vi "Mirao52e.vi"() -> ()   [LabVIEW 2011]
panel:
  in  "?":enum32{"Main", "Debug"}(tab)
  in  "Flat Shape File Path":string="FLAT_MIRAO_0229_01.mro"
  out "error out":errorcluster
  out "flat":dbl[](array[numeric])
  out "received":dbl[](array[numeric])
  out "SyncString":string
  in  "Debug":bool
  out "# messages received":u64
  out "DM response":i8
  out "open return value":i8
  in  "stop":bool
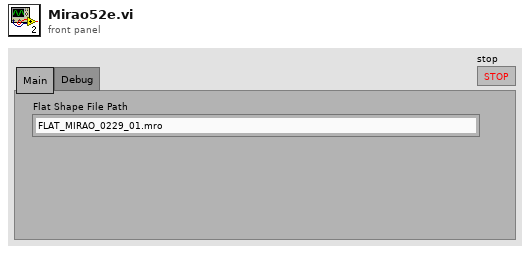
[diagram p1: front panel]
types:
  T1 = enum32{"invalid app kind", "Development System", "Run Time System", "Student Edition", "Embedded LabVIEW", "Evaluation", "Custom"}
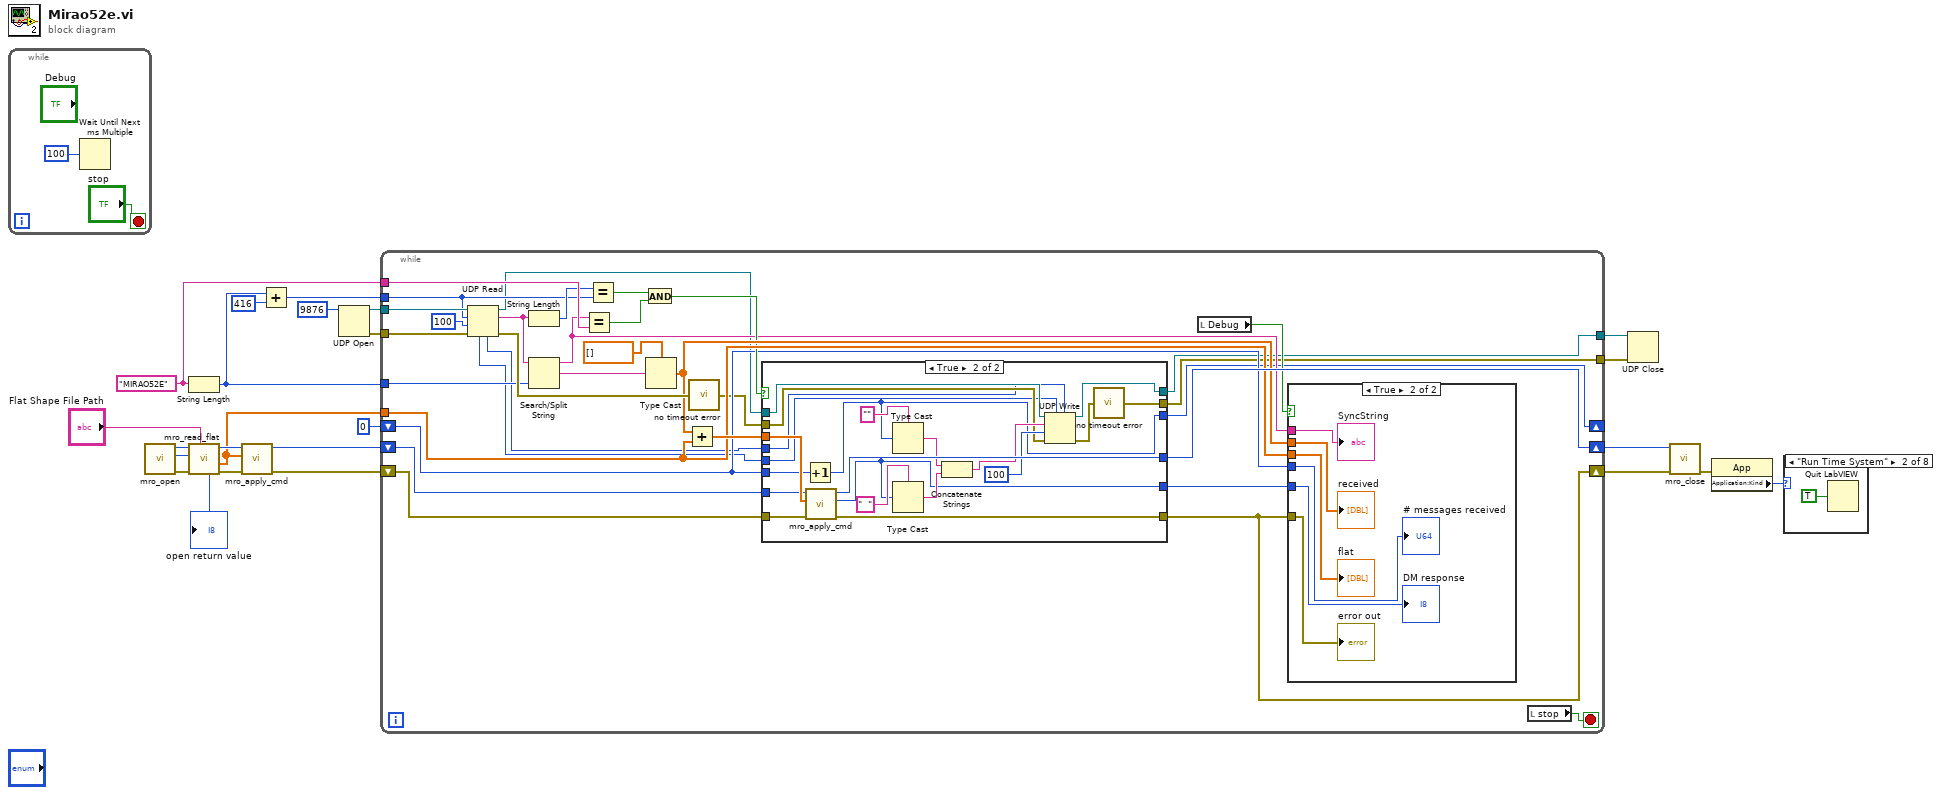
[diagram p0: block diagram]
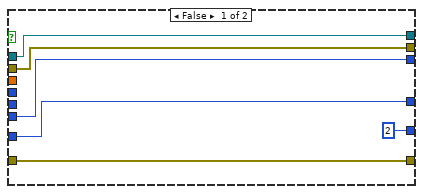
[diagram p10: hidden frame]
diagram:
  w2 = "MIRAO52E" ("data out")
  n1 = while {
    stop <- "stop" stop-if-true
    n2 = Wait Until Next ms Multiple(millisecond multiple=u32 100) -> ()  [unwired: 1 out]
  }
  n3 = call "mro_open.vi"() -> ("error out"=w21:errorcluster, "return type"=→"open return value":i8, "status"=w23:i32)  [unwired: 9 in]
  n4 = String Length(string=w2) -> (length=w3:i32)
  n5 = call "mro_read_flat.vi"("FilePath"="Flat Shape File Path", "error in (no error)"=w21, "status in"=w23) -> ("error out"=w11:errorcluster, "flat"=w9:dbl[], "status out"=w13:i32)  [unwired: 5 in, 1 out]
  n6 = call "mro_apply_cmd.vi"("error in (no error)"=w11, "command"=w9, "status in"=w13) -> ("error out"=w10:errorcluster, "status out"=w12:i32)  [unwired: 6 in, 1 out]
  n7 = Add(x=w3, y=416 ("max size (548)")) -> (x+y=w4:i32)
  n8 = UDP Open(11:u16 9876 ("Port")) -> (port=w20:refnum<k16>, 0:w19:errorcluster)  [unwired: 4 in, 1 out]
  n9 = while {
    tunnel: w9 -> [w48]
    tunnel: w20 -> [w57]
    tunnel: w19 -> [w56]
    tunnel: [w29] -> w18
    tunnel: [w30] -> w17
    shift-right: [w58] -> w22
    shift-left: w12 -> [w52]
    shift-right: [w41] -> w8
    shift-left: w10 -> [w51]
    shift-right: [w33] -> _
    shift-left: u64 0 ("Port") -> [w34]
    tunnel: w4 -> [w42]
    tunnel: w3 -> [w40]
    tunnel: w2 -> [w47]
    stop <- w35 stop-if-true
    n10 = UDP Read(connection ID=w57, max size (548)=w42, timeout ms (25000)=100, 8:w56) -> (data out=w39:string, error out=w54:errorcluster, 3:w28:refnum<k16>, 4:w26:u16, 6:w27:u32)
    n11 = String Length(string=w39) -> (length=w43:i32)
    n12 = Search/Split String(string=w39, offset (0)=w40) -> (substring before match=w38:string, match + rest of string=w37:string)  [unwired: 1 in, 1 out]
    n13 = Equal?(x=w38, y=w47) -> (x = y?=w45:bool)
    n14 = Equal?(x=w43, y=w42) -> (x = y?=w44:bool)
    n15 = And(x=w44, y=w45) -> (x .and. y?=w46:bool)
    n16 = Type Cast(type=dbl[] [] ("command"), x=w37) -> (*(type *) &x=w49:dbl[])
    n17 = Add(x=w49, y=w48) -> (x+y=w50:dbl[])
    n18 = call "no timeout error.vi"("error in (no error)"=w54) -> ("error out"=w31:errorcluster)
    n19 = case shown="True" w46 {
      tunnel: [w69 w91] -> w58
      tunnel: [w70 w90] -> w41
      tunnel: w50 -> [_ w89]
      tunnel: w52 -> [w69 w88]
      tunnel: w51 -> [w70 w87]
      tunnel: w34 -> [w68 w86]
      tunnel: [w68 w74] -> w33
      tunnel: [i8 2 ("return type") w73] -> w32
      tunnel: w31 -> [w65 w78]
      tunnel: [w65 w77] -> w30
      tunnel: [w66 w76] -> w29
      tunnel: w28 -> [w66 w75]
      tunnel: w27 -> [_ w72]
      tunnel: w26 -> [_ w71]
      frame False {
      }
      frame True {
        n20 = Increment(x=w86) -> (x+1=w74:u64)
        n21 = call "mro_apply_cmd.vi"("error in (no error)"=w87, "command"=w89, "status in"=w88) -> ("error out"=w90:errorcluster, "return type"=w73:i8, "status out"=w91:i32)  [unwired: 6 in]
        n22 = Type Cast(type="", x=w74) -> (*(type *) &x=w84:string)
        n23 = Type Cast(type="  ", x=w73) -> (*(type *) &x=w83:string)
        n24 = Concatenate Strings(w84, w83) -> (w79:string)
        n25 = UDP Write(address=w72, port or service name=w71, connection ID=w75, data in=w79, 8:w78, 9:100 ("timeout ms (25000)")) -> (error out=w80:errorcluster, 3:w76:refnum<k16>)
        n26 = call "no timeout error.vi"("error in (no error)"=w80) -> ("error out"=w77:errorcluster)
      }
    }
    n27 = local read "Debug"() -> (w36:bool)
    n28 = case shown="True" w36 {
      tunnel: w49 -> [_ w64]
      tunnel: w48 -> [_ w63]
      tunnel: w38 -> [_ w62]
      tunnel: w41 -> [_ w61]
      tunnel: w34 -> [_ w60]
      tunnel: w32 -> [_ w59]
      frame False {
      }
      frame True {
        "flat" <- w63
        "received" <- w64
        "SyncString" <- w62
        "error out" <- w61
        "# messages received" <- w60
        "DM response" <- w59
      }
    }
    n29 = local read "stop"() -> (w35:bool)
  }
  n30 = UDP Close(connection ID=w18, 8:w17) -> ()  [unwired: 2 out]
  n31 = call "mro_close.vi"("error in (no error)"=w8, "status in"=w22) -> ("error out"=w6:errorcluster)  [unwired: 7 in, 2 out]
  n32 = property class="App"(error in=w6) -> ("Application:Kind"=w7:T1)  [unwired: 1 in, 2 out]
  n33 = case shown="\"Run Time System\"" w7 {
    frame Default {
    }
    frame "Run Time System" {
      n34 = Quit LabVIEW(quit? (T)=TRUE) -> ()
    }
    frame "Student Edition" {
    }
    frame "Embedded LabVIEW" {
    }
    frame "Evaluation" {
    }
    frame "Custom" {
    }
    frame "Development System" {
    }
    frame "invalid app kind" {
    }
  }
